vi "File Operation.vi"(7 "Action (0: Copy)":enum16{"Copy", "Move", "Delete"}(ring), 8 "error in (no error)":errorcluster, 9 "Destination":string, 10 "Source File":string, 11 "VISA resource name":refnum<visa-resource-name>) -> (0 "error out":errorcluster, 3 "VISA resource name out":refnum<visa-resource-name>)   [LabVIEW 2013, in "AWG.lvlib" / "Agilent 3352X Series.lvlib"]
doc: "File operations in file system stored in non-volatile memory ( the instrument memory or an external USB memory)\nInclude move, copy and delete."
uses:
  Agilent 3352X Series.lvlib
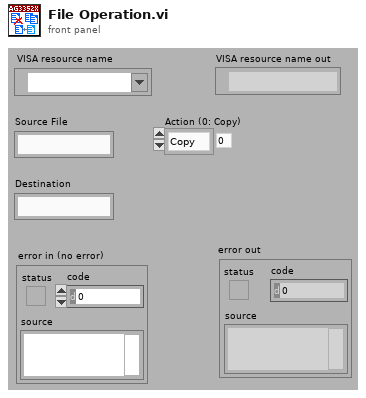
[diagram p1: front panel]
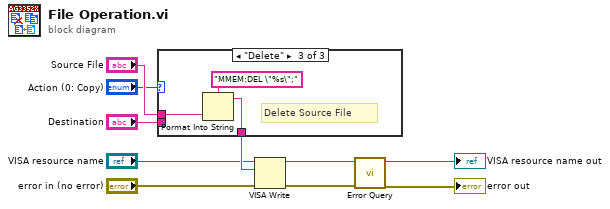
[diagram p0: block diagram]
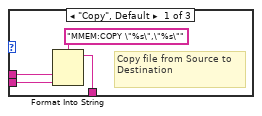
[diagram p2: hidden frame]
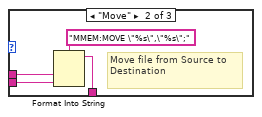
[diagram p3: hidden frame]
diagram:
  n1 = case shown="\"Delete\"" "Action (0: Copy)" {
    tunnel: "Source File" -> [w13 w17 w20]
    tunnel: "Destination" -> [w12 w16 _]
    tunnel: [w11 w15 w19] -> w8
    frame "Copy", Default {
      # "Copy file from Source to Destination"
      n2 = Format Into String(format string="MMEM:COPY \"%s\",\"%s\"", w13, w12) -> (resulting string=w11:string)  [unwired: 2 in, 1 out]
    }
    frame "Move" {
      # "Move file from Source to Destination"
      n3 = Format Into String(format string="MMEM:MOVE \"%s\",\"%s\";", w17, w16) -> (resulting string=w15:string)  [unwired: 2 in, 1 out]
    }
    frame "Delete" {
      # "Delete Source File"
      n4 = Format Into String(format string="MMEM:DEL \"%s\";", w20) -> (resulting string=w19:string)  [unwired: 2 in, 1 out]
    }
  }
  n5 = VISA Write(VISA resource name="VISA resource name", write buffer=w8, error in (no error)="error in (no error)") -> (VISA resource name out=w5:refnum<visa-resource-name>, error out=w4:errorcluster)  [unwired: 1 out]
  n6 = call "Error Query.vi"("error in (no error)"=w4, "VISA resource name"=w5) -> ("error out"=→"error out":errorcluster, "VISA resource name out"=→"VISA resource name out":refnum<visa-resource-name>)  [unwired: 8 out]
